vi "Drive Straight (SubVI).vi"() -> ()   [LabVIEW 2014]
panel:
  out "Left Drive Value":dbl
  out "Right Drive Value":dbl
  in  "Left Joystick Value":dbl
  in  "Right Joystick Value":dbl
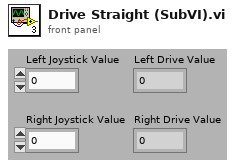
[diagram p1: front panel]
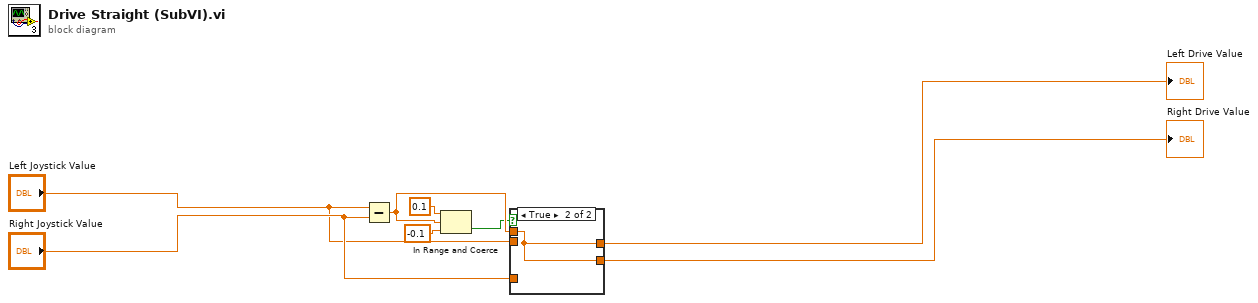
[diagram p0: block diagram]
diagram:
  n1 = Subtract(x="Left Joystick Value", y="Right Joystick Value") -> (x-y=w6:dbl)
  n2 = In Range and Coerce(upper limit=0.1, x=w6, lower limit=-0.1) -> (In Range?=w3:bool)  [unwired: 1 out]
  n3 = case shown="True" w3 {
    tunnel: [w10 w11] -> w4
    tunnel: [w9 w11] -> w5
    tunnel: w6 -> [_ w11]
    tunnel: "Left Joystick Value" -> [w10 _]
    tunnel: "Right Joystick Value" -> [w9 _]
    frame False {
    }
    frame True {
    }
  }
  "Right Drive Value" <- w5
  "Left Drive Value" <- w4
